vi "UIRef.vi"(8 "error in":errorcluster, 11 "Fgen Instrument":refnum<class "Fgen Instrument.lvclass">) -> (0 "error out":errorcluster, 2 "VI refnum":refnum<vi>, 3 "Fgen Instrument out":refnum<class "Fgen Instrument.lvclass">)   [LabVIEW 2025, in "Fgen.lvlib" / "Fgen Instrument.lvclass"]
doc: "Copyright 2017 National Instruments Corporation\n\nLicensed under the Apache License, Version 2.0 (the \"License\"); you may not use this file except in compliance with the License. You may obtain a copy of the License at http://www.apache.org/licenses/LICENSE-2.0\nUnless required by applicable law or agreed to in writing, software distributed under the License is distributed on an \"AS IS\" BASIS, WITHOUT WARRANTIES OR CONDITIONS OF ANY KIND, either express or implied. See the License for the specific language governing permissions and limitations under the License."
uses:
  Fgen Instrument.lvclass
  Fgen Instrument UI.vi
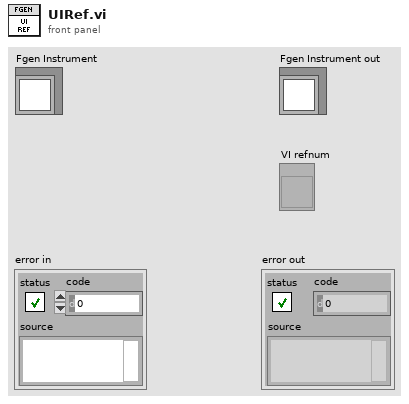
[diagram p1: front panel]
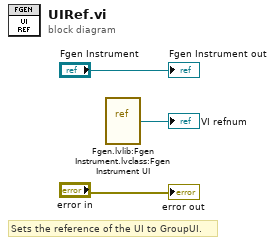
[diagram p0: block diagram]
diagram:
  # "Sets the reference of the UI to GroupUI."
  n1 = vi-ref "Fgen.lvlib:Fgen Instrument.lvclass:Fgen Instrument UI.vi"() -> (→"VI refnum":refnum<vi>)
  "error out" <- "error in"
  "Fgen Instrument out" <- "Fgen Instrument"
